vi "Configure Hardware Piezo.vi"(8 "error in (no error)":errorcluster, 11 "Hardware Configuration in":T1) -> (0 "error out":errorcluster, 3 "Hardware Configuration out":T1)   [LabVIEW 2013, in "Piezo.lvlib"]
uses:
  Piezo/Piezo.lvlib
  Hardware Configuration Piezo.ctl
  <vilib>/DAQmx/create/channels.llb/DAQmx Create Channel (AI-Voltage-Basic).vi
  <vilib>/DAQmx/configure/timing.llb/DAQmx Timing (Sample Clock).vi
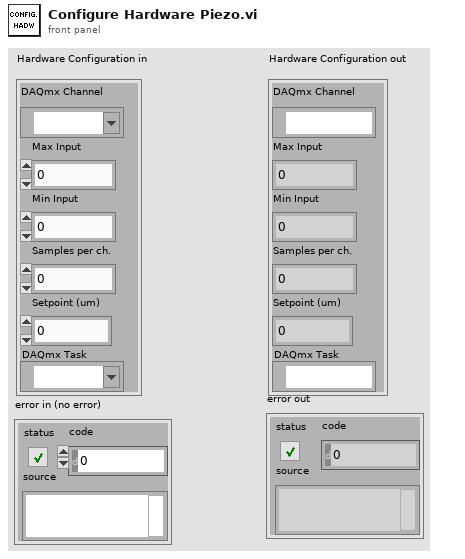
[diagram p1: front panel]
types:
  T1 = typedef "Piezo.lvlib/Hardware Configuration Piezo.ctl" = cluster{"DAQmx Channel":tag, "Max Input":dbl, "Min Input":dbl, "Samples per ch.":dbl, "Setpoint (um)":dbl, "DAQmx Task":refnum<k21>}
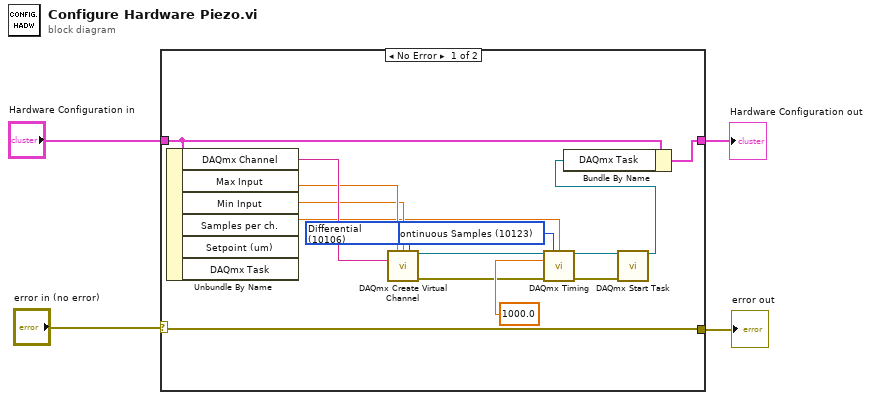
[diagram p0: block diagram]
diagram:
  n1 = case shown="No Error" "error in (no error)" {
    selector: "error in (no error)" -> [w8 w21]
    tunnel: [w8 w21] -> w3
    tunnel: "Hardware Configuration in" -> [w7 w20]
    tunnel: [w5 w20] -> w1
    frame No Error {
      w16 = 10123 items=["Finite Samples"=10178, "Continuous Samples"=10123, "Hardware Timed Single Point"=12522] ("sample mode")
      w19 = 10106 items=["default"=-1, "RSE"=10083, "NRSE"=10078, "Differential"=10106, "Pseudodifferential"=12529] ("input terminal configuration")
      n2 = Unbundle By Name(w7) -> ("DAQmx Channel"=w12:tag, "Max Input"=w11:dbl, "Min Input"=w10:dbl, "Samples per ch."=w9:dbl)  [unwired: 2 out]
      n3 = call-poly <vilib>:"DAQmx Create Virtual Channel.vi"("maximum value"=w11, "minimum value"=w10, "input terminal configuration"=w19, "physical channels"=w12) -> ("task out"=w18:refnum<k21>, "error out"=w14:errorcluster)  [unwired: 10 in]
      n4 = call-poly <vilib>:"DAQmx Timing.vi"("task/channels in"=w18, "sample mode"=w16, "samples per channel"=w9, "rate"=1000.0, "error in"=w14) -> ("task out"=w17:refnum<k21>, "error out"=w13:errorcluster)  [unwired: 9 in]
      n5 = call <vilib>:"DAQmx Start Task.vi"("task/channels in"=w17, "error in"=w13) -> ("task out"=w6:refnum<k21>)  [unwired: 12 in, 1 out]
      n6 = Bundle By Name(cluster=w7, "DAQmx Task"=w6) -> (w5:T1)
    }
    frame Error {
    }
  }
  "Hardware Configuration out" <- w1
  "error out" <- w3
